vi "Configure Control AI Range(GS Sqrt).vi"(0 "VISA resource name":refnum<visa-resource-name>, 1 "Unit No. (0)":i32 min=0 max=6, 2 "Range, Span, Bias":T3={"GS Range (0 : 1-5V)"=0, "Enable Span (False)"=FALSE, "Lower Span (-2.0000)"=-2.0, "Upper Span (2.0000)"=2.0, "Bias (0)"=0.0} {"Upper Span (2.0000)" min=-99999.0 max=99999.0 step=1.0 format="%_5g"; "Lower Span (-2.0000)" min=-99999.0 max=99999.0 step=1.0 format="%_5g"; "GS Range (0 : 1-5V)" items=["1-5V", "0.4-2V"]}, 3 "Scaling":T2={"Floating point position (2)"=2, "Lower Scaling (0)"=0.0, "Upper Scaling (100.00)"=100.0, "Unit Character (\"\")"=""} {"Upper Scaling (100.00)" format="%_6g"; "Lower Scaling (0)" format="%_6g"; "Floating point position (2)" min=0 max=5 step=1}, 4 "Module No.(0)":i32 min=0 max=9, 5 "AI No.(1)":i32=1 min=1 max=2, 6 "Low cut":T1 {"Output (0: Zero)" items=["Zero", "Linear"]; "Low-cut (0.0)" min=0.0 max=5.0 step=0.1 format="%.1g"}, 7 "error in (no error)":errorcluster) -> (20 "VISA resource name out":refnum<visa-resource-name>, 21 "AI No.":i32, 24 "Unit No.":i32, 25 "Module No.":i32, 27 "error out":errorcluster)   [LabVIEW 2020, in "Yokogawa GX Series.lvlib"]
doc: "Set GS Sqrt range of AI channel in PID module.\n\nCommand: SCtrlRangeAI"
uses:
  <instrlib>/Yokogawa GX Series/Yokogawa GX Series.lvlib
  <instrlib>/Yokogawa GX Series/Private/GS Range.vi
panel:
  # "%"
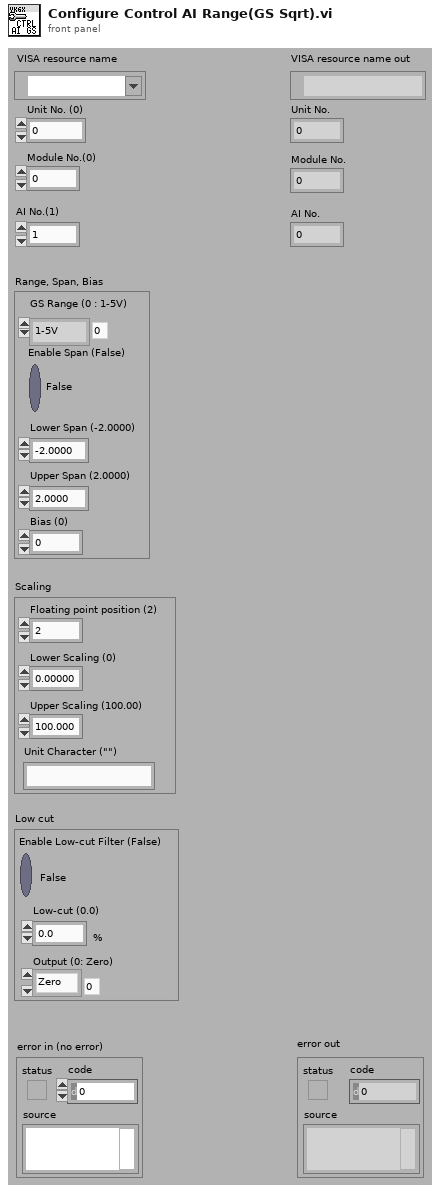
[diagram p1: front panel]
types:
  T1 = cluster{"Enable Low-cut Filter (False)":bool, "Low-cut (0.0)":dbl, "Output (0: Zero)":u16}
  T2 = cluster{"Floating point position (2)":i32, "Lower Scaling (0)":dbl, "Upper Scaling (100.00)":dbl, "Unit Character (\"\")":string}
  T3 = cluster{"GS Range (0 : 1-5V)":i32, "Enable Span (False)":bool, "Lower Span (-2.0000)":dbl, "Upper Span (2.0000)":dbl, "Bias (0)":dbl}
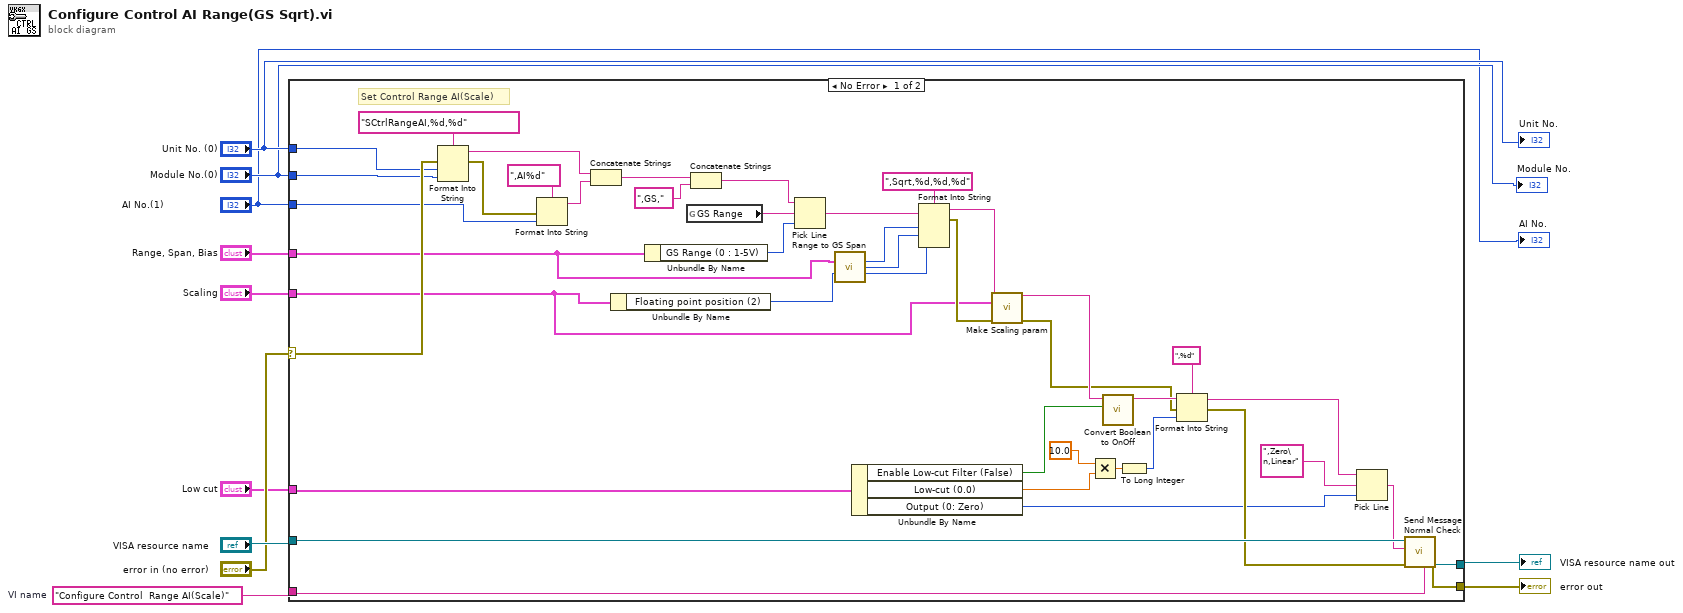
[diagram p0: block diagram]
diagram:
  w7 = "Configure Control  Range AI(Scale)"  # VI name
  n1 = case shown="No Error" "error in (no error)" {
    selector: "error in (no error)" -> [w50 w55]
    tunnel: [w54 w56] -> w11
    tunnel: [w53 w55] -> w10
    tunnel: "VISA resource name" -> [w52 w56]
    tunnel: w7 -> [w49 _]
    tunnel: "Unit No. (0)" -> [w48 _]
    tunnel: "Module No.(0)" -> [w47 _]
    tunnel: "AI No.(1)" -> [w45 _]
    tunnel: "Range, Span, Bias" -> [w28 _]
    tunnel: "Scaling" -> [w27 _]
    tunnel: "Low cut" -> [w16 _]
    frame No Error {
      # "Set Control Range AI(Scale)"
      n2 = Format Into String(format string="SCtrlRangeAI,%d,%d", error in=w50, w48, w47) -> (resulting string=w43:string, error out=w44:errorcluster)  [unwired: 1 in]
      n3 = Format Into String(format string=",AI%d", error in=w44, w45) -> (resulting string=w42:string)  [unwired: 1 in, 1 out]
      n4 = Concatenate Strings(w43, w42) -> (w37:string)
      n5 = Unbundle By Name(w27) -> ("Floating point position (2)"=w29:i32)
      n6 = Unbundle By Name(w28) -> ("GS Range (0 : 1-5V)"=w40:i32)
      n7 = global read "GS Range.vi" "GS Range"() -> (w38:string)
      n8 = Concatenate Strings(w37, ",GS,") -> (w41:string)
      n9 = Pick Line(string ("")=w41, multi-line string=w38, line index=w40) -> (output string=w30:string)
      n10 = call <instrlib>:"Range to GS Span.vi"("Range and span"=w28, "Floating Point Position (2)"=w29) -> ("Lower Span"=w35:i32, "Upper Span"=w34:i32, "Bias"=w33:i32)  [unwired: 11 in]
      n11 = Unbundle By Name(w16) -> ("Enable Low-cut Filter (False)"=w21:bool, "Low-cut (0.0)"=w20:dbl, "Output (0: Zero)"=w13:u16)
      n12 = Format Into String(format string=",Sqrt,%d,%d,%d", initial string=w30, w35, w34, w33) -> (resulting string=w32:string, error out=w31:errorcluster)  [unwired: 1 in]
      n13 = call <instrlib>:"Make Scaling param.vi"("String (\"\")"=w32, "Scaling"=w27, "error in (no error)"=w31) -> ("String After"=w19:string, "error out"=w18:errorcluster)  [unwired: 11 in]
      n14 = Multiply(x=10.0, y=w20) -> (x*y=w23:dbl)
      n15 = call <instrlib>:"Convert Boolean to OnOff.vi"("On/Off"=w21, "Initial String (\"\")"=w19) -> ("Resulting String"=w26:string)  [unwired: 9 in]
      n16 = To Long Integer(number=w23) -> (32bit integer=w22:i32)
      n17 = Format Into String(format string=",%d", initial string=w26, error in=w18, w22) -> (resulting string=w14:string, error out=w17:errorcluster)
      n18 = Pick Line(string ("")=w14, multi-line string=",Zero\n,Linear", line index=w13) -> (output string=w12:string)
      n19 = call <instrlib>:"Send Message Normal Check.vi"("Source (\"\")"=w49, "error in (no error)"=w17, "Send Message (\"\")"=w12, "VISA resource name"=w52) -> ("error out"=w53:errorcluster, "VISA resource name out"=w54:refnum<visa-resource-name>)  [unwired: 2 in, 4 out]
    }
    frame Error {
    }
  }
  "error out" <- w10
  "VISA resource name out" <- w11
  "Unit No." <- "Unit No. (0)"
  "Module No." <- "Module No.(0)"
  "AI No." <- "AI No.(1)"
